vi "get Active Object Transform.vi"(11 "Scene in":refnum<class "Scene.lvclass">) -> (3 "Transform":T1)   [LabVIEW 2020, in "Scene.lvclass"]
uses:
  Scene.lvclass
  Scene.lvclass/Scene.ctl
  Graphics/Libraries/3D/Vector 3D.ctl
  Graphics/Libraries/3D/3D.lvlib
  Graphics/Libraries/3D/Transform.ctl
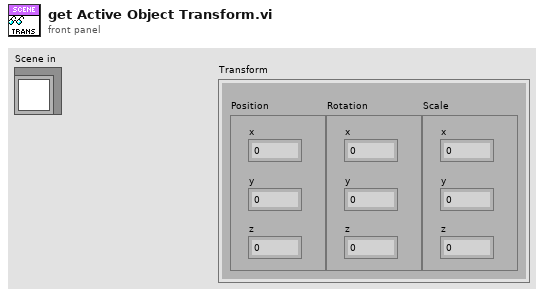
[diagram p1: front panel]
types:
  T1 = typedef "3D.lvlib/Transform.ctl" = cluster{"Position":T2, "Rotation":T2, "Scale":T2}
  T2 = typedef "3D.lvlib/Vector 3D.ctl" = cluster{"x":sgl, "y":sgl, "z":sgl}
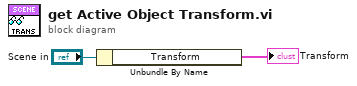
[diagram p0: block diagram]
diagram:
  n1 = Unbundle By Name("Scene in") -> ("Transform"=→"Transform":T1)
